vi "GetDecayForLifetimeImage.vi"(0 "channel":u8=1, 2 "F2-channel":u8=1, 3 "Array 2":i32[](array[numeric]), 4 "micro times":u16[](array[numeric]), 7 "empty decay":u32[][](array[numeric]), 8 "router":u8[](array[numeric]), 9 "Array":bool[](array[boolean])) -> (1 "lifetime [ns]":ext[](array[numeric]) format="%.2f", 5 "F2-value":dbl[](array[numeric]) format="%.2f")   [LabVIEW 2009]
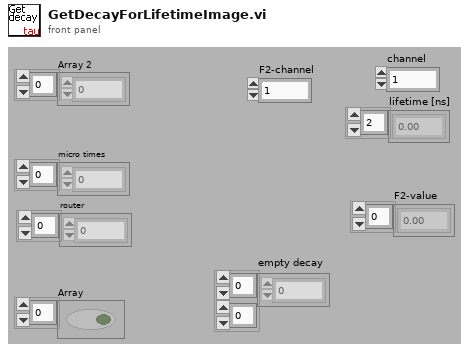
[diagram p1: front panel]
types:
  T1 = typedef "spotproperties.ctl" = cluster{"draw?":bool, "plane":u32, "Coordinates":i32[], "TACWindow":cluster{"TACWindow1":i32, "TACWindow2":i32}, "Lifetime[ns]":ext[], "tauerror":dbl[], "F2-Value overall":dbl, "overall intensity":u32[], "F2-Value TAC":dbl, "TAC intensity":u32[], "Decay":u32[][]}
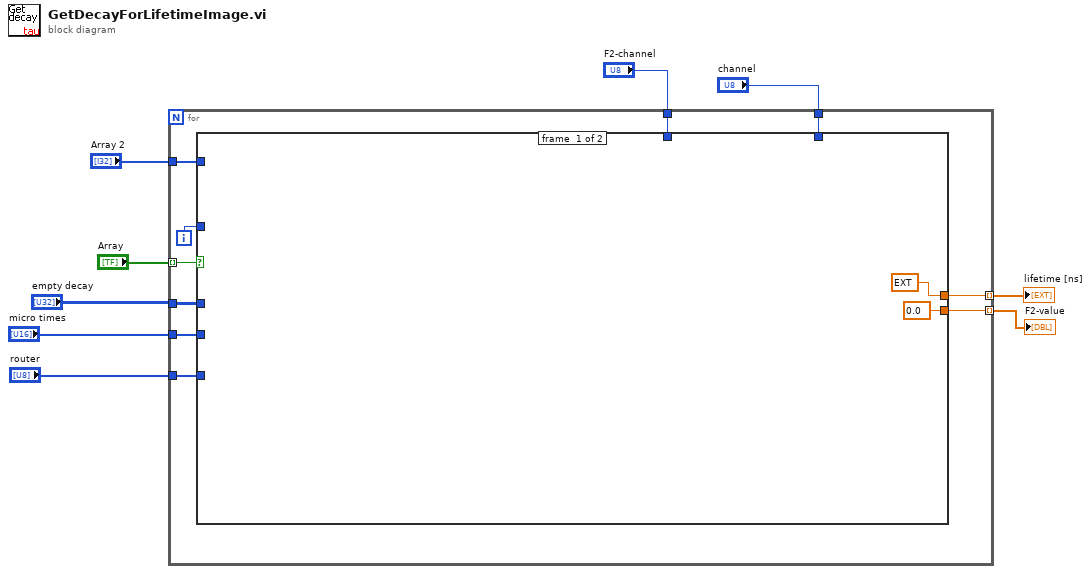
[diagram p0: block diagram]
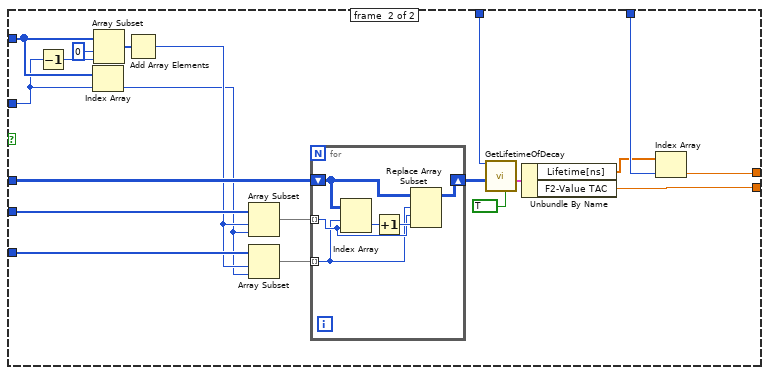
[diagram p2: hidden frame]
diagram:
  n1 = for {
    tunnel: "Array 2" -> [w17]
    tunnel: "Array" -> [w18] mode=indexing
    tunnel: "micro times" -> [w19]
    tunnel: "router" -> [w15]
    tunnel: "empty decay" -> [w14]
    tunnel: "F2-channel" -> [w13]
    tunnel: [w12] -> w4 mode=indexing
    tunnel: [w11] -> w3 mode=indexing
    tunnel: "channel" -> [w10]
    i -> [w16]
    n2 = case shown="True" w18 {
      tunnel: w19 -> [_ w41]
      tunnel: w17 -> [_ w32]
      tunnel: w16 -> [_ w29]
      tunnel: w15 -> [_ w40]
      tunnel: w14 -> [_ w37]
      tunnel: w13 -> [_ w35]
      tunnel: [ext 0.0 ("fit tau") w22] -> w12
      tunnel: [0.0 ("F2-Value TAC") w34] -> w11
      tunnel: w10 -> [_ w24]
      frame #0 {
      }
      frame #1 {
        n3 = Decrement(x=w29) -> (x-1=w31:i32)
        n4 = Index Array(array=w32, index=w29) -> (element=w27:i32)
        n5 = Array Subset(array=w32, index=0, length=w31) -> (w33:i32[])
        n6 = Add Array Elements(numeric array=w33) -> (sum=w28:i32)
        n7 = Array Subset(array=w41, index=w28, length=w27) -> (w39:u16[])
        n8 = Array Subset(array=w40, index=w28, length=w27) -> (w38:u8[])
        n9 = for {
          tunnel: w39 -> [w43] mode=indexing
          tunnel: w38 -> [w42] mode=indexing
          shift-right: [w44] -> w26
          shift-left: w37 -> [w45]
          n10 = Index Array(array=w45, index (row)=w42, index (col)=w43) -> (element=w46:u32)
          n11 = Increment(x=w46) -> (x+1=w47:u32)
          n12 = Replace Array Subset(array=w45, new element=w47, index (row)=w42, index (col)=w43) -> (w44:u32[][])
        }
        n13 = call "GetLifetimeOfDecay.vi"("F2-channel"=w35, "decay"=w26, "tauimage"=TRUE) -> ("SpotProperties"=w25:T1)  [unwired: 6 in]
        n14 = Unbundle By Name(w25) -> ("Lifetime[ns]"=w23:ext[], "F2-Value TAC"=w34:dbl)
        n15 = Index Array(array=w23, index=w24) -> (element=w22:ext)
      }
    }
  }
  "lifetime [ns]" <- w4
  "F2-value" <- w3
